vi "Set Data.vi"(10 "Persistent":T1={"Path"=path "", "Select Option?"=TRUE, "Explorer Option?"=TRUE, "Recurse?"=TRUE, "Allow New?"=FALSE, "Filter"="*.*"}, 11 "Static Path Selector in":refnum<class "MGI Static Path Selector.lvclass">) -> (3 "Static Path Selector out":refnum<class "MGI Static Path Selector.lvclass">)   [LabVIEW 2020, in "MGI Static Path Selector.lvclass"]
doc: "Sets the private data as specified."
uses:
  <userlib>/_MGI/User Interface/Path Selector XControl/Class Hierarchy/Static File Selector/MGI Static Path Selector.lvclass
  <userlib>/_MGI/User Interface/Path Selector XControl/Class Hierarchy/Static File Selector/Persistent Data Cluster.ctl
  <userlib>/_MGI/User Interface/Path Selector XControl/Class Hierarchy/Static File Selector/MGI Static Path Selector.lvclass/MGI Static Path Selector.ctl
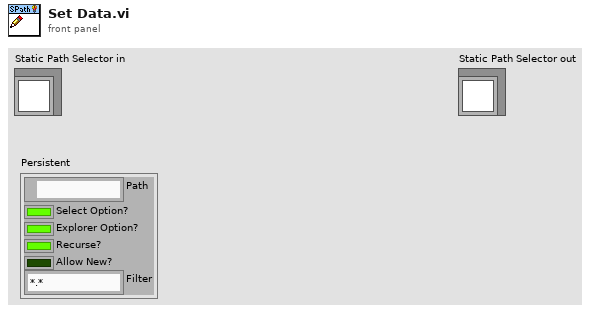
[diagram p1: front panel]
types:
  T1 = typedef "MGI Static Path Selector.lvclass/Persistent Data Cluster.ctl" = cluster{"Path":path, "Select Option?":bool, "Explorer Option?":bool, "Recurse?":bool, "Allow New?":bool, "Filter":string}
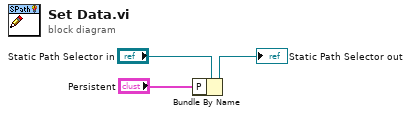
[diagram p0: block diagram]
diagram:
  n1 = Bundle By Name(cluster="Static Path Selector in", "P"="Persistent") -> (→"Static Path Selector out":refnum<class "MGI Static Path Selector.lvclass">)
